vi "atividade 4 ((ajustarrr 10 02.vi"() -> ()   [LabVIEW 2020]
uses:
  <vilib>/Waveform/WDTFileIO.llb/Export Waveforms To Spreadsheet File (1D).vi
panel:
  out "Waveform Chart":waveform(dbl)(graph)
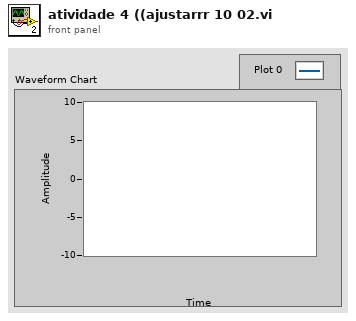
[diagram p1: front panel]
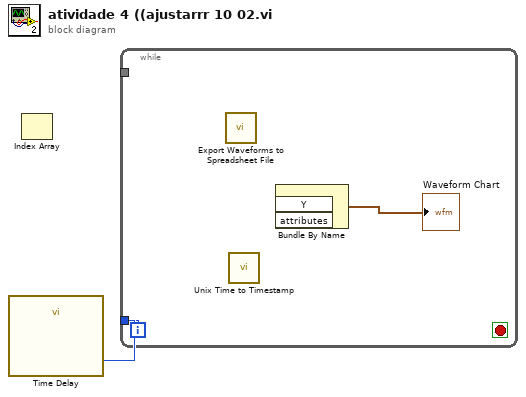
[diagram p0: block diagram]
diagram:
  n1 = Index Array "Index Array"() -> ()  [unwired: 2 in, 1 out]
  n2 = while {
    tunnel: [_] -> w2
    tunnel: [w3] -> w1
    i -> [w3]
    stop <- _ stop-if-true
    n3 = call-poly <vilib>:"Export Waveforms to Spreadsheet File.vi"() -> ()  [unwired: 10 in, 2 out]
    n4 = call <vilib>:"Unix Time to Timestamp.vi"() -> ()  [unwired: 10 in, 2 out]
    n5 = Bundle By Name() -> (→"Waveform Chart":waveform(dbl))  [unwired: 3 in]
  }
  n6 = call "Time Delay"("Delay Time (s)"=w1) -> ()  [unwired: 10 in, 1 out]
